vi "InterpolateCompensationCoefficients.vi"(0 "fs (Hz)":dbl, 1 "SignalLength":i32, 2 "Apply Phase Correction?":bool=TRUE, 4 "F-CompArray":dbl[][](array[numeric])) -> (3 "Frequencies":dbl[](array[numeric])=[1.0, 0.9893, 1.019, 1.0269, 1.0344, 1.0416, 1.0487, 1.0558, 1.0628, 1.0701, 1.0776, 1.0854, 1.0937, 1.1026, 1.1121, 1.1224, 1.1336, 1.1457, 1.1589, 1.1733, 1.189, 1.2061, 1.2246, 1.2447, 1.2662, 1.289, 1.3129, 1.3376, 1.3632, 1.3892, 1.4157, 1.4425, 1.4693, 1.496, 1.5226, 1.5491, 1.5754, 1.6016, 1.6277, 1.6535, 1.6792, 1.7046, 1.7298, 1.7548, 1.7794, 1.8033, 1.8263, 1.8483, 1.869, 1.8882, 1.9058, 1.9215, 1.935, 1.9464, 1.9556, 1.9628, 1.9684, 1.9723, 1.9748, 1.9762, 1.9765, 1.9759, 1.9748, 1.9731, 1.9711, 1.9689, 1.9667, 1.9646, 1.9628, 1.9614, 1.9606, 1.9605, 1.9612, 1.963, 1.9657, 1.9693, 1.9738, 1.979, 1.9848, 1.9913, 1.9983, 2.0059, 2.0138, 2.0221, 2.0308, 2.0401, 2.05, 2.0607, 2.0722, 2.0847, 2.0983, 2.113, 0.0, 0.0, 0.0, 0.0, 0.0, 0.0, 0.0, 0.0, 0.0, 0.0, 0.0, 0.0, 0.0, 0.0, 0.0, 0.0, 0.0, 0.0, 0.0, 0.0, 0.0, 0.0, 0.0, 0.0, 0.0, 0.0, 0.0, 0.0, 0.0, 0.0, 0.0, 0.0, 0.0, 0.0, 0.0, 0.0, 0.0, 0.0, 0.0, 0.0, 0.0, 0.0, 0.0, 0.0, 0.0, 0.0, 0.0, 0.0, 0.0, 0.0, 0.0, 0.0], 5 "InterpolatedPhase":dbl[](array[numeric])=[1.0, 0.9893, 1.019, 1.0269, 1.0344, 1.0416, 1.0487, 1.0558, 1.0628, 1.0701, 1.0776, 1.0854, 1.0937, 1.1026, 1.1121, 1.1224, 1.1336, 1.1457, 1.1589, 1.1733, 1.189, 1.2061, 1.2246, 1.2447, 1.2662, 1.289, 1.3129, 1.3376, 1.3632, 1.3892, 1.4157, 1.4425, 1.4693, 1.496, 1.5226, 1.5491, 1.5754, 1.6016, 1.6277, 1.6535, 1.6792, 1.7046, 1.7298, 1.7548, 1.7794, 1.8033, 1.8263, 1.8483, 1.869, 1.8882, 1.9058, 1.9215, 1.935, 1.9464, 1.9556, 1.9628, 1.9684, 1.9723, 1.9748, 1.9762, 1.9765, 1.9759, 1.9748, 1.9731, 1.9711, 1.9689, 1.9667, 1.9646, 1.9628, 1.9614, 1.9606, 1.9605, 1.9612, 1.963, 1.9657, 1.9693, 1.9738, 1.979, 1.9848, 1.9913, 1.9983, 2.0059, 2.0138, 2.0221, 2.0308, 2.0401, 2.05, 2.0607, 2.0722, 2.0847, 2.0983, 2.113, 0.0, 0.0, 0.0, 0.0, 0.0, 0.0, 0.0, 0.0, 0.0, 0.0, 0.0, 0.0, 0.0, 0.0, 0.0, 0.0, 0.0, 0.0, 0.0, 0.0, 0.0, 0.0, 0.0, 0.0, 0.0, 0.0, 0.0, 0.0, 0.0, 0.0, 0.0, 0.0, 0.0, 0.0, 0.0, 0.0, 0.0, 0.0, 0.0, 0.0, 0.0, 0.0, 0.0, 0.0, 0.0, 0.0, 0.0, 0.0, 0.0, 0.0, 0.0, 0.0], 6 "InterpolatedCoefficients":dbl[](array[numeric])=[1.0, 0.9893, 1.019, 1.0269, 1.0344, 1.0416, 1.0487, 1.0558, 1.0628, 1.0701, 1.0776, 1.0854, 1.0937, 1.1026, 1.1121, 1.1224, 1.1336, 1.1457, 1.1589, 1.1733, 1.189, 1.2061, 1.2246, 1.2447, 1.2662, 1.289, 1.3129, 1.3376, 1.3632, 1.3892, 1.4157, 1.4425, 1.4693, 1.496, 1.5226, 1.5491, 1.5754, 1.6016, 1.6277, 1.6535, 1.6792, 1.7046, 1.7298, 1.7548, 1.7794, 1.8033, 1.8263, 1.8483, 1.869, 1.8882, 1.9058, 1.9215, 1.935, 1.9464, 1.9556, 1.9628, 1.9684, 1.9723, 1.9748, 1.9762, 1.9765, 1.9759, 1.9748, 1.9731, 1.9711, 1.9689, 1.9667, 1.9646, 1.9628, 1.9614, 1.9606, 1.9605, 1.9612, 1.963, 1.9657, 1.9693, 1.9738, 1.979, 1.9848, 1.9913, 1.9983, 2.0059, 2.0138, 2.0221, 2.0308, 2.0401, 2.05, 2.0607, 2.0722, 2.0847, 2.0983, 2.113, 0.0, 0.0, 0.0, 0.0, 0.0, 0.0, 0.0, 0.0, 0.0, 0.0, 0.0, 0.0, 0.0, 0.0, 0.0, 0.0, 0.0, 0.0, 0.0, 0.0, 0.0, 0.0, 0.0, 0.0, 0.0, 0.0, 0.0, 0.0, 0.0, 0.0, 0.0, 0.0, 0.0, 0.0, 0.0, 0.0, 0.0, 0.0, 0.0, 0.0, 0.0, 0.0, 0.0, 0.0, 0.0, 0.0, 0.0, 0.0, 0.0, 0.0, 0.0, 0.0])   [LabVIEW 2016]
uses:
  <vilib>/gmath/NI_Gmath.lvlib
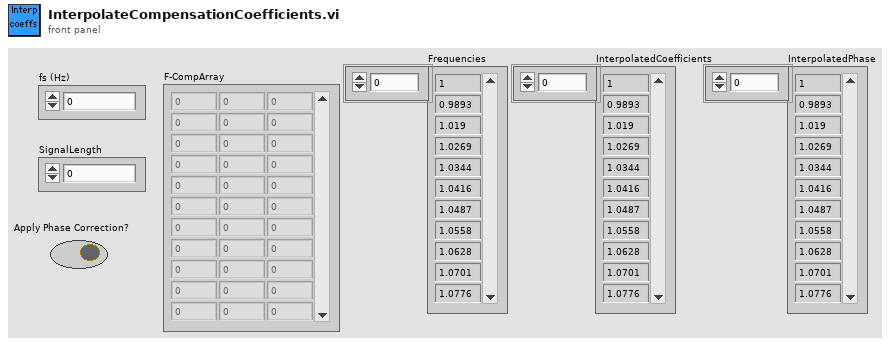
[diagram p1: front panel]
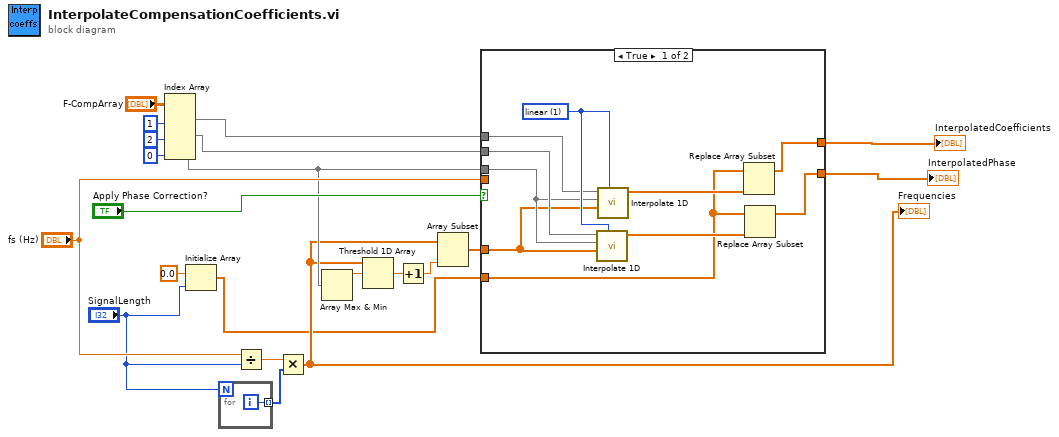
[diagram p0: block diagram]
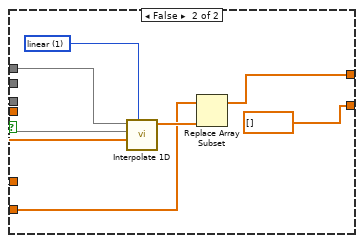
[diagram p2: hidden frame]
diagram:
  n1 = Index Array(array="F-CompArray", index (col) #1=1 ("disabled index (col)"), index (col) #2=2 ("index (col)"), index (col) #3=0 ("disabled index (col)")) -> (element #1=w4:dbl[], element #2=w15:dbl[], element #3=w8:dbl[])  [unwired: 3 in]
  n2 = Initialize Array(0.0 ("element"), "SignalLength") -> (w1:dbl[])
  n3 = for {
    N: "SignalLength" -> [_]
    tunnel: [w22] -> w11 mode=indexing
    i -> [w22]
  }
  n4 = Divide(x="fs (Hz)", y="SignalLength") -> (x/y=w10:dbl)
  n5 = Multiply(x=w10, y=w11) -> (x*y=w7:dbl[])
  "Frequencies" <- w7
  n6 = Array Max & Min(array=w8) -> (max value=w12:dbl)  [unwired: 3 out]
  n7 = Threshold 1D Array(2:w12, 3:w7) -> (0:w13:dbl)  [unwired: 1 in]
  n8 = Increment(x=w13) -> (x+1=w14:dbl)
  n9 = Array Subset(array=w7, length=w14) -> (w6:dbl[])  [unwired: 1 in]
  n10 = case shown="True" "Apply Phase Correction?" {
    tunnel: "fs (Hz)" -> [_ _]
    tunnel: [w30 w34] -> w20
    tunnel: [w28 dbl[] [] ("yi")] -> w19
    tunnel: w4 -> [w27 w38]
    tunnel: w15 -> [w26 _]
    tunnel: w8 -> [w25 w37]
    tunnel: w6 -> [w24 w36]
    tunnel: w1 -> [w23 w33]
    frame True {
      w32 = 1 items=["nearest", "linear", "spline", "cubic Hermite", "Lagrange"] ("method")
      n11 = call <vilib>:"Interpolate 1D.vi"("method"=w32, "xi"=w24, "X"=w25, "Y"=w26) -> ("yi"=w29:dbl[])  [unwired: 2 in, 5 out]
      n12 = call <vilib>:"Interpolate 1D.vi"("method"=w32, "xi"=w24, "X"=w25, "Y"=w27) -> ("yi"=w31:dbl[])  [unwired: 2 in, 5 out]
      n13 = Replace Array Subset(array=w23, new element=w31) -> (w30:dbl[])  [unwired: 1 in]
      n14 = Replace Array Subset(array=w23, new element=w29) -> (w28:dbl[])  [unwired: 1 in]
    }
    frame False {
      w40 = 1 items=["nearest", "linear", "spline", "cubic Hermite", "Lagrange"] ("method")
      n15 = call <vilib>:"Interpolate 1D.vi"("method"=w40, "xi"=w36, "X"=w37, "Y"=w38) -> ("yi"=w35:dbl[])  [unwired: 2 in, 5 out]
      n16 = Replace Array Subset(array=w33, new element=w35) -> (w34:dbl[])  [unwired: 1 in]
    }
  }
  "InterpolatedCoefficients" <- w20
  "InterpolatedPhase" <- w19
